vi "Resize Window.vi"(7 "reference":refnum<vi>, 10 "Height":i16) -> (0 "error out":errorcluster)   [LabVIEW 2015]
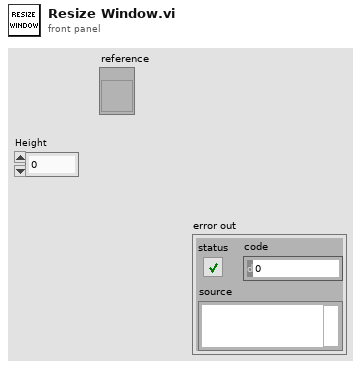
[diagram p1: front panel]
types:
  T1 = typedef "LVRectTypeDef.ctl" = cluster{"Left":i16, "Top":i16, "Right":i16, "Bottom":i16}
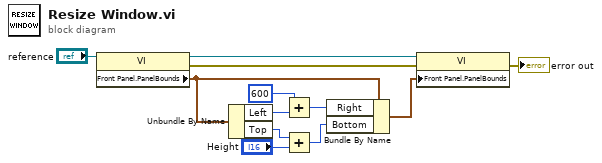
[diagram p0: block diagram]
diagram:
  n1 = property class="VI"(reference="reference") -> (reference out=w2:refnum<vi>, error out=w11:errorcluster, "Front Panel.PanelBounds"=w7:T1)  [unwired: 1 in]
  n2 = Unbundle By Name(w7) -> ("Left"=w10:i16, "Top"=w9:i16)
  n3 = Add(x=i16 600, y=w10) -> (x+y=w6:i16)
  n4 = Add(x=w9, y="Height") -> (x+y=w5:i16)
  n5 = Bundle By Name(cluster=w7, "Right"=w6, "Bottom"=w5) -> (w4:T1)
  n6 = property class="VI"(reference=w2, error in=w11, "Front Panel.PanelBounds"=w4) -> (error out=→"error out":errorcluster)  [unwired: 1 out]
